vi "Get gRPC Service Methods.vi"(8 "error in (no error)":errorcluster, 11 "Service ref in":u64) -> (0 "error out":errorcluster, 2 "Service Methods":u64[](array[numeric]), 3 "Service ref out":u64)   [LabVIEW 2019, in "gRPC Template Creation Utility.lvlib"]
uses:
  gRPC Template Creation Utility.lvlib
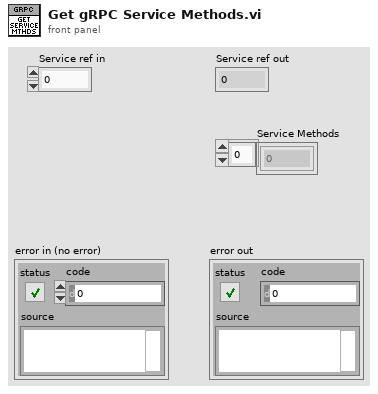
[diagram p1: front panel]
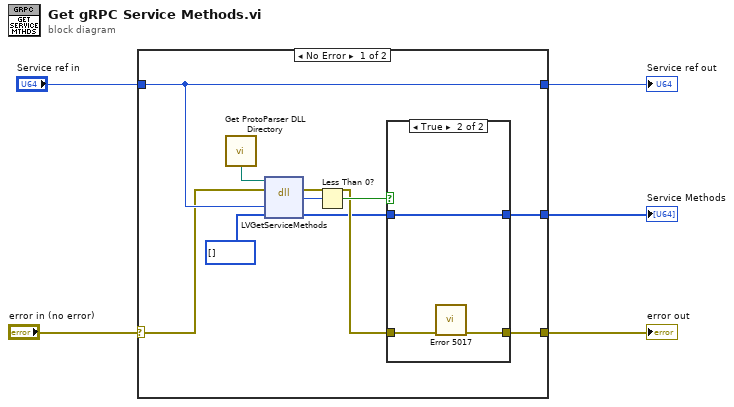
[diagram p0: block diagram]
diagram:
  n1 = case shown="No Error" "error in (no error)" {
    selector: "error in (no error)" -> [w12 w21]
    tunnel: [w6 _] -> w5
    tunnel: "Service ref in" -> [w13 w22]
    tunnel: [w13 w22] -> w2
    tunnel: [w8 w21] -> w1
    frame No Error {
      n2 = call "Get ProtoParser DLL Directory.vi"() -> ("Proto Parser Directory"=w14:path)
      n3 = dll-call lib="C:/Users/XEnderMD/Desktop/LV gRPC/labview source/gRPC Scripting Tools/Proto Parser API/dll/labview_grpc_generator.dll" fn="LVGetServiceMethods"(path in=w14, error in=w12, "service"=w13, "serviceMethods"=u64[] []) -> (error out=w9:errorcluster, "return type"=w11:i32, "serviceMethods"=w7:u64[])  [unwired: 2 in, 1 out]
      n4 = Less Than 0?(x=w11) -> (x < 0?=w10:bool)
      n5 = case shown="True" w10 {
        tunnel: w9 -> [w16 w20]
        tunnel: [w16 w19] -> w8
        tunnel: w7 -> [w17 w18]
        tunnel: [w17 w18] -> w6
        frame False {
        }
        frame True {
          n6 = call "Error 5017.vi"("error in (no error)"=w20) -> ("error out"=w19:errorcluster)  [unwired: 10 in]
        }
      }
    }
    frame Error {
    }
  }
  "Service Methods" <- w5
  "Service ref out" <- w2
  "error out" <- w1
